vi "Read Show value tip.vi"(9 "NumericWithScale in":refnum<class "NumericWithScale.lvclass">) -> (3 "NumericWithScale out":refnum<class "NumericWithScale.lvclass">, 4 "Show value tip":bool)   [LabVIEW 2014, in "Raspberry Pi Compatible Compiler for LabVIEW.lvlib" / "NumericWithScale.lvclass"]
uses:
  NumericWithScale.lvclass
  NumericWithScale.lvclass/NumericWithScale.ctl
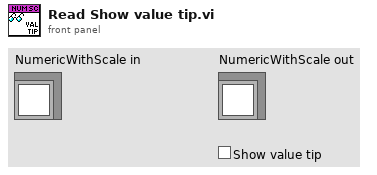
[diagram p1: front panel]
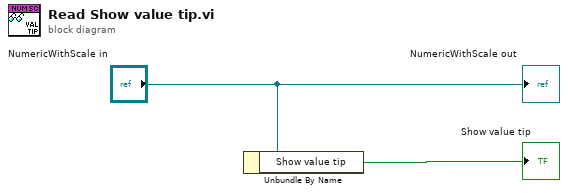
[diagram p0: block diagram]
diagram:
  n1 = Unbundle By Name("NumericWithScale in") -> ("Show value tip"=→"Show value tip":bool)
  "NumericWithScale out" <- "NumericWithScale in"
